vi "Config.vi"(8 "error in (no error)":errorcluster, 10 "Setting":variant, 11 "Chroma 19020":refnum<class "Chroma 190020.lvclass">) -> (0 "error out":errorcluster, 3 "Chroma 19020 out":refnum<class "Chroma 190020.lvclass">)   [LabVIEW 2025, in "HiPOT.lvlib" / "Chroma 190020.lvclass"]
uses:
  Chroma 190020.lvclass
  C:/Users/Public/Documents/Sandia National Labs/TSS Plugin/CEF.lvlibp/Node/CEF_Node.lvclass
  C:/Working copy/tss/Plugin/Engines/HiPOT/HiPOT Instrument/HiPOT Instrument.lvclass
  C:/Users/Public/Documents/Sandia National Labs/TSS Plugin/Abstract Engine.lvlibp/Plugin/Abstract/Abstract Instrument/Abstract Instrument.lvclass
  HiPOT configuration/HiPOT configuration.lvclass
  Chroma 190020.lvclass/Chroma 190020.ctl
  HiPOT configuration/HiPOT configuration.lvclass/HiPOT configuration.ctl
  HiPOT Channel/HiPOT Channel.lvclass
  HiPOT Channel configuration/HiPOT Channel configuration.lvclass
  C:/Users/Public/Documents/Sandia National Labs/TSS Plugin/Abstract Engine.lvlibp/Plugin/Abstract/Channel configuration/Channel configuration.lvclass
  Users/Public/Documents/Sandia National Labs/TSS Plugin/Abstract Engine.lvlibp/Plugin/Abstract/Abstract Instrument/Channel.ctl
  HiPOT configuration/Read ACIR Setting.vi
  Users/Public/Documents/Sandia National Labs/TSS Plugin/CEF.lvlibp/Node/ReadChildren.vi
  Users/Public/Documents/Sandia National Labs/TSS Plugin/Abstract Engine.lvlibp/Plugin/Abstract/Channel configuration/Read Channel Setting.vi
  Users/Public/Documents/Sandia National Labs/TSS Plugin/CEF.lvlibp/Node/CEF_Node.lvclass
  Users/Public/Documents/Sandia National Labs/TSS Plugin/CEF.lvlibp/serializable configuration/CEF_serializable configuration.lvclass
  Users/Public/Documents/Sandia National Labs/TSS Plugin/Abstract Engine.lvlibp/Plugin/Abstract/Abstract Instrument/Abstract Instrument.lvclass
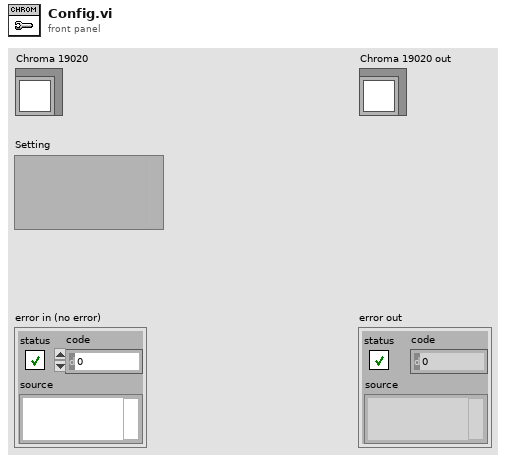
[diagram p1: front panel]
types:
  T1 = typedef "Abstract Engine.lvlibp/Abstract Instrument.lvclass/Channel.ctl" = cluster{"Alias":string, "DataType":enum16{"Anaolg Input", "Waveform"}, "Unit":enum16{"---", "V", "A", "Ohm", "Hz", "uF", "degC", "deg"}, "Upper limit":dbl, "Lower limit":dbl, "Measurement":variant}
  T2 = typedef "Abstract Engine.lvlibp/Channel configuration.lvclass/Default Channel.ctl" = cluster{"Address":string, "SW Alias":string, "Enabled":bool, "Type":string, "Description":string}
  T3 = typedef "HiPOT.lvlib/HiPOT configuration.lvclass/HiPOT Instrument Setting.ctl" = cluster{"DC Voltage":dbl, "High Limit":dbl, "Test Time(s)":u32}
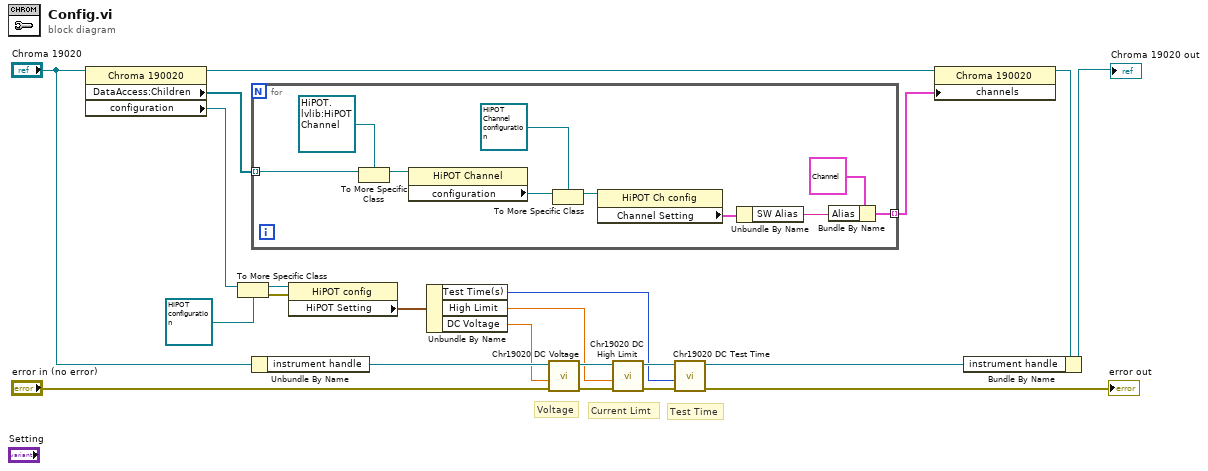
[diagram p0: block diagram]
diagram:
  # "Current Limt"
  # "Test Time"
  # "Voltage"
  n1 = property class="Chroma 190020"(reference="Chroma 19020") -> (reference out=w19:refnum<class "Chroma 190020.lvclass">, "DataAccess:Children"=w3:refnum<data-value>[], "configuration"=w4:refnum<class "CEF_serializable configuration.lvclass">)  [unwired: 1 in, 1 out]
  n2 = To More Specific Class(target class=refnum<class "HiPOT configuration.lvclass"> refnum ("Digitizer.lvlib:Digitizer configuration.lvclass"), reference=w4) -> (specific class reference=w20:refnum<class "HiPOT configuration.lvclass">, error out=w7:errorcluster)  [unwired: 1 in]
  n3 = for {
    tunnel: w3 -> [w32] mode=indexing
    tunnel: [w23] -> w1 mode=indexing
    n4 = To More Specific Class(target class=refnum<data-value> refnum ("data value reference"), reference=w32) -> (specific class reference=w30:refnum<data-value>)  [unwired: 1 in, 1 out]
    n5 = property class="HiPOT Channel"(reference=w30) -> ("configuration"=w29:refnum<class "CEF_serializable configuration.lvclass">)  [unwired: 1 in, 2 out]
    n6 = To More Specific Class(target class=refnum<class "HiPOT Channel configuration.lvclass"> refnum ("HiPOT.lvlib:HiPOT Channel config"), reference=w29) -> (specific class reference=w27:refnum<class "HiPOT Channel configuration.lvclass">)  [unwired: 1 in, 1 out]
    n7 = property class="HiPOT Ch config"(reference=w27) -> ("Channel Setting"=w26:T2)  [unwired: 1 in, 2 out]
    n8 = Unbundle By Name(w26) -> ("SW Alias"=w25:string)
    n9 = Bundle By Name(cluster=T1 {"Alias"="ch0", "DataType"=enum."Anaolg Input", "Unit"=enum."V", "Upper limit"=10.0, "Lower limit"=-10.0, "Measurement"=variant(dbl 0.0)} ("Channel"), "Alias"=w25) -> (w23:T1)
  }
  n10 = Unbundle By Name("Chroma 19020") -> ("instrument handle"=w13:refnum<k15>)
  n11 = property class="HiPOT config"(reference=w20, error in=w7) -> ("HiPOT Setting"=w8:T3)  [unwired: 2 out]
  n12 = Unbundle By Name(w8) -> ("Test Time(s)"=w11:u32, "High Limit"=w10:dbl, "DC Voltage"=w9:dbl)
  n13 = call <instrlib>:"Chr19020 DC Voltage.vi"("error in (no error)"="error in (no error)", "dc voltage"=w9, "instrument handle"=w13) -> ("error out"=w16:errorcluster, "instrument handle out"=w15:refnum<k15>)  [unwired: 7 in]
  n14 = call <instrlib>:"Chr19020 DC High Limit.vi"("error in (no error)"=w16, "high limit"=w10, "instrument handle"=w15) -> ("error out"=w18:errorcluster, "instrument handle out"=w17:refnum<k15>)  [unwired: 7 in]
  n15 = call <instrlib>:"Chr19020 DC Test Time.vi"("error in (no error)"=w18, "test time"=w11, "instrument handle"=w17) -> ("error out"=→"error out":errorcluster, "instrument handle out"=w12:refnum<k15>)  [unwired: 7 in]
  n16 = property class="Chroma 190020"(reference=w19, "channels"=w1) -> (reference out=w2:refnum<class "Chroma 190020.lvclass">)  [unwired: 1 in, 1 out]
  n17 = Bundle By Name(cluster=w2, "instrument handle"=w12) -> (→"Chroma 19020 out":refnum<class "Chroma 190020.lvclass">)
